vi "StringParser.vi"(1 "String":string) -> (0 "array":string[](array[string]))   [LabVIEW 2014]
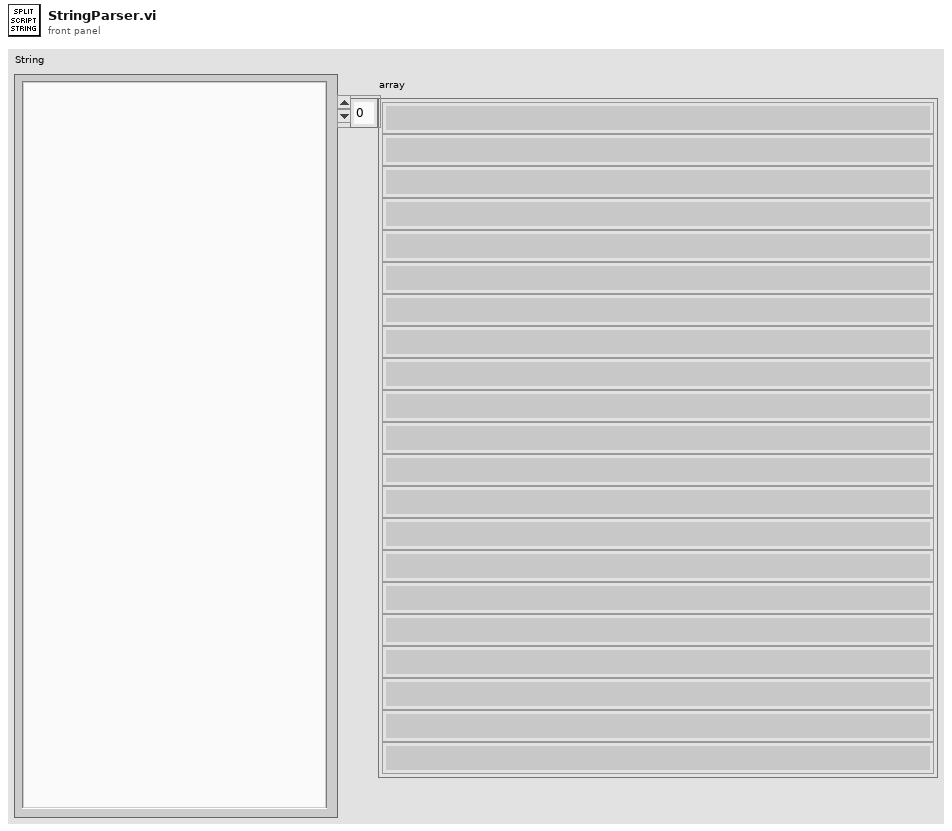
[diagram p1: front panel]
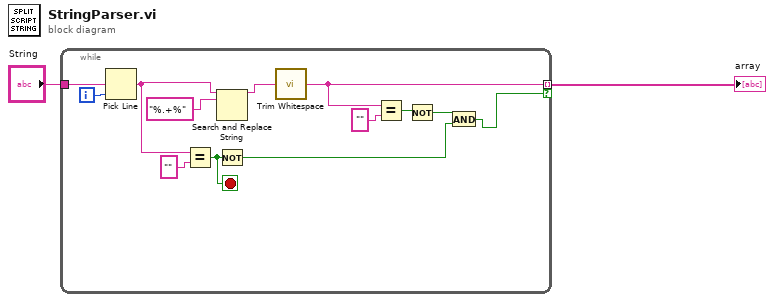
[diagram p0: block diagram]
diagram:
  n1 = while {
    tunnel: "String" -> [w15]
    tunnel: [w7] -> w1 mode=indexing if=w3
    i -> [w14]
    stop <- w12 stop-if-true
    n2 = Pick Line(multi-line string=w15, line index=w14) -> (output string=w10:string)  [unwired: 1 in]
    n3 = Equal?(x=w10, y="") -> (x = y?=w12:bool)
    n4 = Search and Replace String(input string=w10, search string="%.+%") -> (result string=w9:string)  [unwired: 6 in, 3 out]
    n5 = Not(x=w12) -> (.not. x?=w4:bool)
    n6 = call <vilib>:"Trim Whitespace.vi"("string"=w9) -> ("trimmed string"=w7:string)  [unwired: 1 in]
    n7 = Equal?(x=w7, y="") -> (x = y?=w6:bool)
    n8 = Not(x=w6) -> (.not. x?=w5:bool)
    n9 = And(x=w5, y=w4) -> (x .and. y?=w3:bool)
  }
  "array" <- w1
